vi "GetDeviceName.vi"(8 "error in (no error)":errorcluster, 11 "SETI_LV_FPGA in":refnum<class "SETI_LV_FPGA.lvclass">) -> (0 "error out":errorcluster, 2 "DEV-NAME":string, 3 "SETI_LV_FPGA out":refnum<class "SETI_LV_FPGA.lvclass">)   [LabVIEW 2015, in "SETI_LV_FPGA.lvclass"]
uses:
  SETI_LV_FPGA.lvclass
  SETI_LV_FPGA.lvclass/SETI_LV_FPGA.ctl
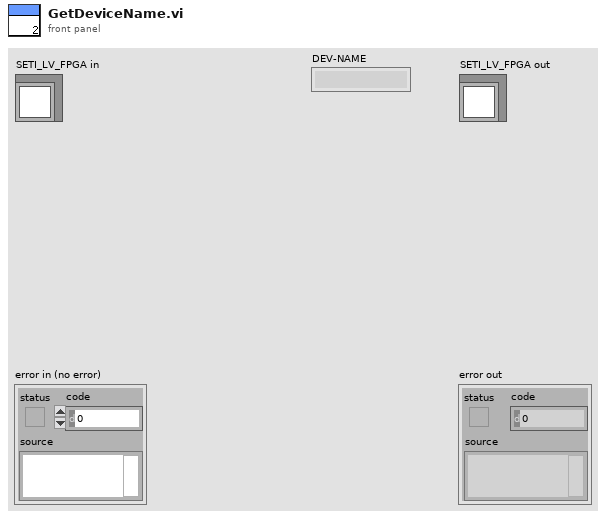
[diagram p1: front panel]
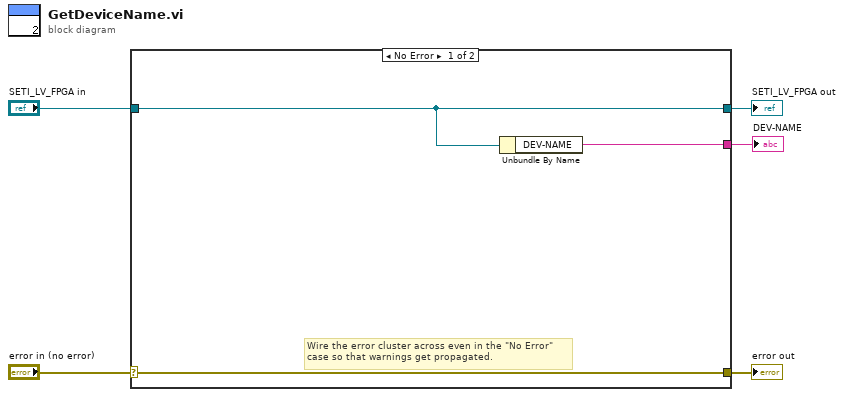
[diagram p0: block diagram]
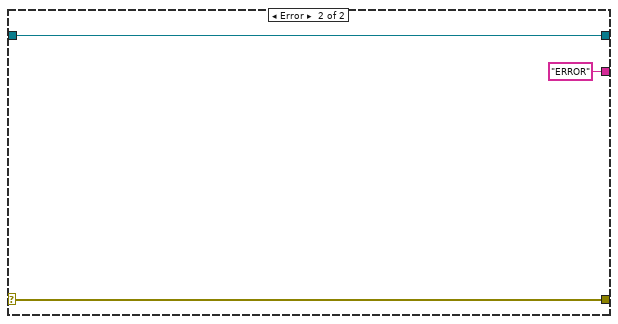
[diagram p2: hidden frame]
diagram:
  n1 = case shown="No Error" "error in (no error)" {
    selector: "error in (no error)" -> [w8 w11]
    tunnel: [w8 w11] -> w4
    tunnel: [w7 w10] -> w2
    tunnel: "SETI_LV_FPGA in" -> [w7 w10]
    tunnel: [w6 "ERROR" ("DEV-NAME")] -> w1
    frame No Error {
      # "Wire the error cluster across even in the \"No Error\"\ncase so that warnings get propagated."
      n2 = Unbundle By Name(w7) -> ("DEV-NAME"=w6:string)
    }
    frame Error {
    }
  }
  "error out" <- w4
  "SETI_LV_FPGA out" <- w2
  "DEV-NAME" <- w1
